vi "Init Analysis Graph.vi"(6 "Z Scale.Marker Values[]":cluster{"Numeric":dbl, "Numeric":u32}[](array[cluster]), 7 "Graphs":T1, 8 "error in (no error)":errorcluster, 9 "Shots":u32, 10 "Image Size":cluster{"Height":u32, "Width":u32}, 11 "Analysis Graph in":refnum<class "Analysis Graph.lvclass">) -> (0 "error out":errorcluster, 3 "Analysis Graph out":refnum<class "Analysis Graph.lvclass">)   [LabVIEW 2023, in "Analysis Graph.lvclass"]
uses:
  Analysis Graph.lvclass
  Analysis Graph.lvclass/Analysis Graph.ctl
  Series Graph/Series Graph.lvclass
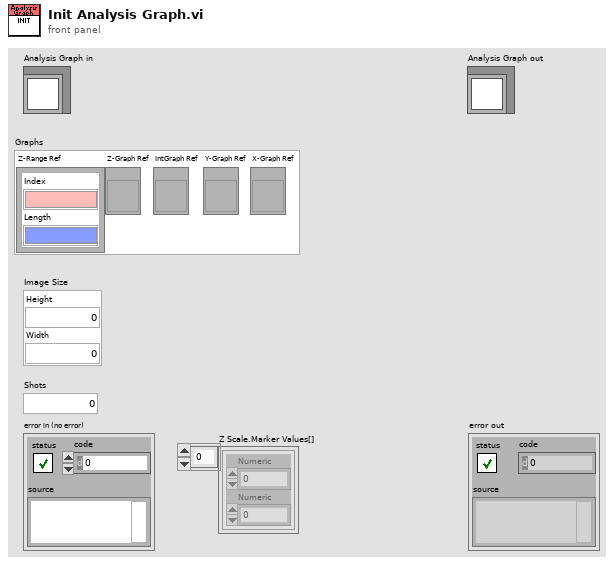
[diagram p1: front panel]
types:
  T1 = cluster{"Z-Range Ref":refnum<vi>, "Z-Graph Ref":refnum<vi>, "IntGraph Ref":refnum<vi>, "Y-Graph Ref":refnum<vi>, "X-Graph Ref":refnum<vi>}
  T2 = cluster{"Z-Graph Ref":refnum<vi>, "IntGraph Ref":refnum<vi>, "Y-Graph Ref":refnum<vi>, "X-Graph Ref":refnum<vi>}
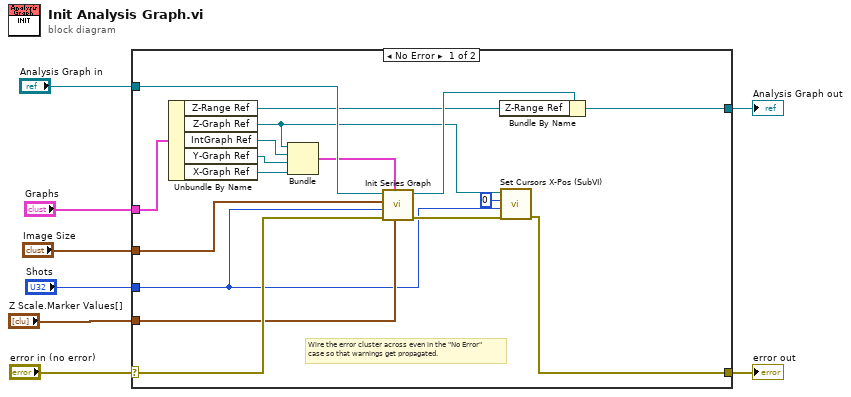
[diagram p0: block diagram]
diagram:
  n1 = case shown="No Error" "error in (no error)" {
    selector: "error in (no error)" -> [w18 w27]
    tunnel: [w12 w27] -> w7
    tunnel: [w15 w26] -> w5
    tunnel: "Analysis Graph in" -> [w25 w26]
    tunnel: "Graphs" -> [w24 _]
    tunnel: "Image Size" -> [w19 _]
    tunnel: "Shots" -> [w11 _]
    tunnel: "Z Scale.Marker Values[]" -> [w17 _]
    frame No Error {
      # "Wire the error cluster across even in the \"No Error\"\ncase so that warnings get propagated."
      n2 = Unbundle By Name(w24) -> ("Z-Range Ref"=w10:refnum<vi>, "Z-Graph Ref"=w9:refnum<vi>, "IntGraph Ref"=w23:refnum<vi>, "Y-Graph Ref"=w22:refnum<vi>, "X-Graph Ref"=w21:refnum<vi>)
      n3 = Bundle("Z-Graph Ref"=w9, "IntGraph Ref"=w23, "Y-Graph Ref"=w22, "X-Graph Ref"=w21) -> (w20:T2)  [unwired: 1 in]
      n4 = call "Init Series Graph.vi"("Z Scale.Marker Values[]"=w17, "Graphs"=w20, "error in (no error)"=w18, "Shots"=w11, "Image Size"=w19, "Series Graph in"=w25) -> ("error out"=w13:errorcluster, "Series Graph out"=w16:refnum<class "Analysis Graph.lvclass">)  [unwired: 4 in]
      n5 = Bundle By Name(cluster=w16, "Z-Range Ref"=w10) -> (w15:refnum<class "Analysis Graph.lvclass">)
      n6 = call "Set Cursors X-Pos (SubVI).vi"("error in (no error)"=w13, "length"=w11, "index"=0, "WaveformGraph in"=w9) -> ("error out"=w12:errorcluster)  [unwired: 7 in]
    }
    frame Error {
    }
  }
  "error out" <- w7
  "Analysis Graph out" <- w5
